vi "Broadcast.vi"   [LabVIEW 2015]
uses:
  Global/Globalclient.vi
types:
  T1 = enum16{"Standard", "Buffered", "CRLF", "Immediate"}
  T2 = typedef "消息头.ctl" = string[]
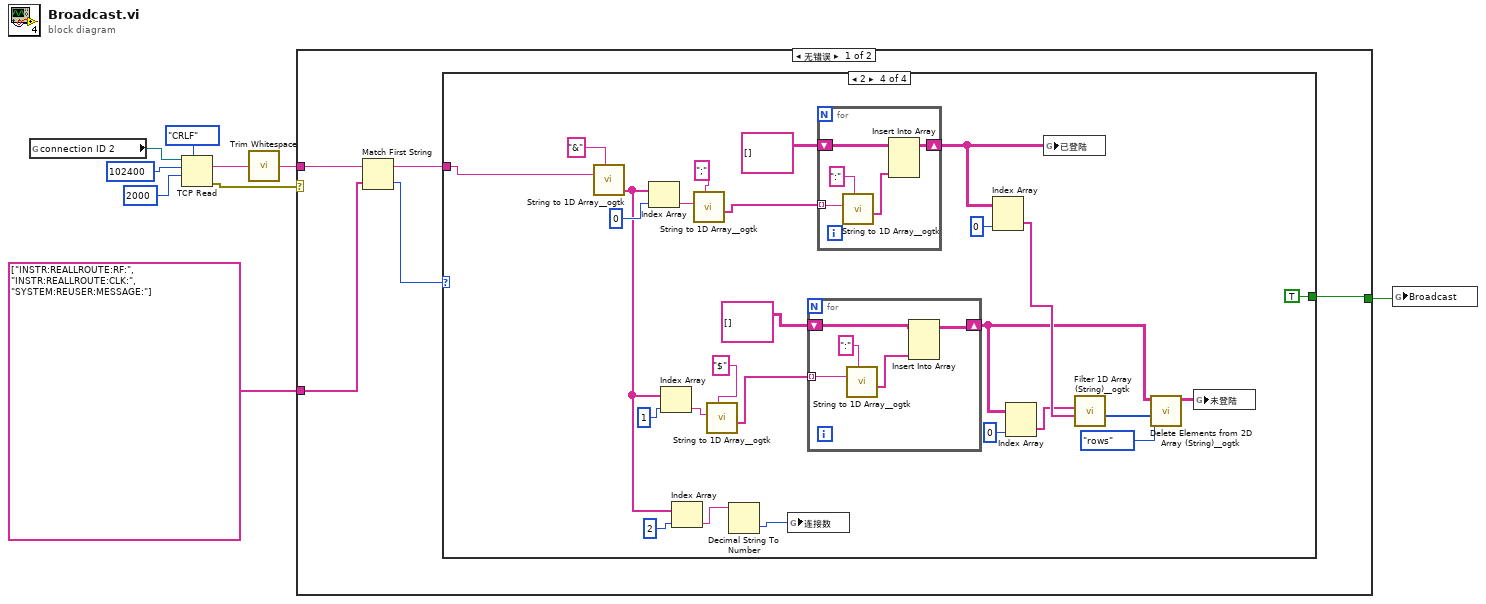
[diagram p0: block diagram]
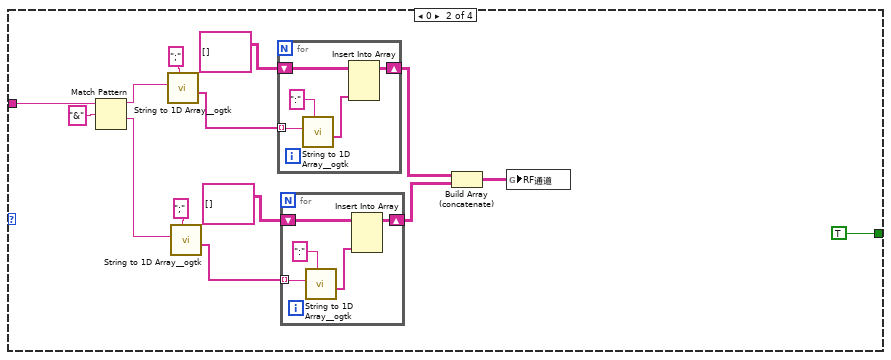
[diagram p3: hidden frame]
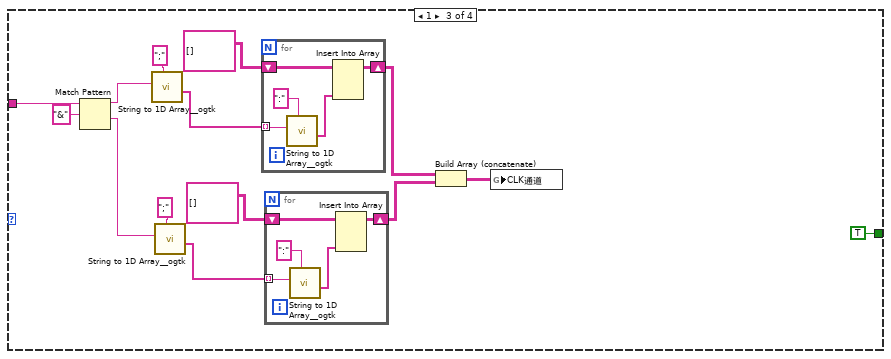
[diagram p4: hidden frame]
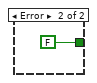
[diagram p5: hidden frame]
diagram:
  n1 = global read "Globalclient.vi" "connection ID 2"() -> (w9:refnum<k5>)
  n2 = TCP Read(connection ID=w9, bytes to read=102400, 7:T1."CRLF" ("mode (standard)"), 9:2000 ("timeout ms (25000)")) -> (data out=w3:string, error out=w4:errorcluster)  [unwired: 1 in, 1 out]
  n3 = call <vilib>:"Trim Whitespace.vi"("string"=w3) -> ("trimmed string"=w2:string)  [unwired: 1 in]
  n4 = case shown="无错误" w4 {
    tunnel: w2 -> [w14 _]
    tunnel: T2 ["INSTR:REALLROUTE:RF:", "INSTR:REALLROUTE:CLK:", "SYSTEM:REUSER:MESSAGE:"] ("消息头") -> [w13 _]
    tunnel: [w10 FALSE] -> w1
    frame No Error {
      n5 = Match First String(2:w13, 3:w14) -> (0:w11:i32, 1:w12:string)
      n6 = case shown="2" w11 {
        tunnel: w12 -> [_ w16 w41 w64]
        tunnel: [_ TRUE TRUE TRUE] -> w10
        frame Default {
        }
        frame 0 {
          n7 = Match Pattern(string=w16, regular expression="&") -> (before substring=w25:string, after substring=w19:string)  [unwired: 1 in, 2 out]
          n8 = call <userlib>:"String to 1D Array__ogtk.vi"("delimiter (Tab)"=";", "string"=w25) -> ("Array of Strings"=w24:string[])  [unwired: 9 in]
          n9 = call <userlib>:"String to 1D Array__ogtk.vi"("delimiter (Tab)"=";", "string"=w19) -> ("Array of Strings"=w21:string[])  [unwired: 9 in]
          n10 = for {
            tunnel: w24 -> [w38] mode=indexing
            shift-right: [w34] -> w18
            shift-left: string[][] [] -> [w36]
            n11 = call <userlib>:"String to 1D Array__ogtk.vi"("delimiter (Tab)"=":", "string"=w38) -> ("Array of Strings"=w35:string[])  [unwired: 9 in]
            n12 = Insert Into Array(array=w36, new element=w35) -> (w34:string[][])  [unwired: 2 in]
          }
          n13 = for {
            tunnel: w21 -> [w33] mode=indexing
            shift-right: [w29] -> w17
            shift-left: string[][] [] -> [w31]
            n14 = call <userlib>:"String to 1D Array__ogtk.vi"("delimiter (Tab)"=":", "string"=w33) -> ("Array of Strings"=w30:string[])  [unwired: 9 in]
            n15 = Insert Into Array(array=w31, new element=w30) -> (w29:string[][])  [unwired: 2 in]
          }
          n16 = Build Array (concatenate)(w18, w17) -> (w28:string[][])
          n17 = global write "Globalclient.vi" "RF通道"(w28) -> ()
        }
        frame 1 {
          n18 = Match Pattern(string=w41, regular expression="&") -> (before substring=w50:string, after substring=w44:string)  [unwired: 1 in, 2 out]
          n19 = call <userlib>:"String to 1D Array__ogtk.vi"("delimiter (Tab)"=";", "string"=w50) -> ("Array of Strings"=w49:string[])  [unwired: 9 in]
          n20 = call <userlib>:"String to 1D Array__ogtk.vi"("delimiter (Tab)"=";", "string"=w44) -> ("Array of Strings"=w46:string[])  [unwired: 9 in]
          n21 = for {
            tunnel: w49 -> [w62] mode=indexing
            shift-right: [w58] -> w43
            shift-left: string[][] [] -> [w60]
            n22 = call <userlib>:"String to 1D Array__ogtk.vi"("delimiter (Tab)"=":", "string"=w62) -> ("Array of Strings"=w59:string[])  [unwired: 9 in]
            n23 = Insert Into Array(array=w60, new element=w59) -> (w58:string[][])  [unwired: 2 in]
          }
          n24 = for {
            tunnel: w46 -> [w57] mode=indexing
            shift-right: [w53] -> w42
            shift-left: string[][] [] -> [w55]
            n25 = call <userlib>:"String to 1D Array__ogtk.vi"("delimiter (Tab)"=":", "string"=w57) -> ("Array of Strings"=w54:string[])  [unwired: 9 in]
            n26 = Insert Into Array(array=w55, new element=w54) -> (w53:string[][])  [unwired: 2 in]
          }
          n27 = Build Array (concatenate)(w43, w42) -> (w40:string[][])
          n28 = global write "Globalclient.vi" "CLK通道"(w40) -> ()
        }
        frame 2 {
          n29 = call <userlib>:"String to 1D Array__ogtk.vi"("delimiter (Tab)"="&", "string"=w64) -> ("Array of Strings"=w70:string[])  [unwired: 9 in]
          n30 = Index Array(array=w70, index=0) -> (element=w79:string)
          n31 = Index Array(array=w70, index=1) -> (element=w75:string)
          n32 = Index Array(array=w70, index=2) -> (element=w68:string)
          n33 = call <userlib>:"String to 1D Array__ogtk.vi"("delimiter (Tab)"=";", "string"=w79) -> ("Array of Strings"=w77:string[])  [unwired: 9 in]
          n34 = call <userlib>:"String to 1D Array__ogtk.vi"("delimiter (Tab)"="$", "string"=w75) -> ("Array of Strings"=w74:string[])  [unwired: 9 in]
          n35 = Decimal String To Number(string=w68) -> (number=w65:i32)  [unwired: 2 in, 1 out]
          n36 = global write "Globalclient.vi" "连接数"(w65) -> ()
          n37 = for {
            tunnel: w74 -> [w93] mode=indexing
            shift-right: [w89] -> w71
            shift-left: string[][] [] -> [w91]
            n38 = call <userlib>:"String to 1D Array__ogtk.vi"("delimiter (Tab)"=":", "string"=w93) -> ("Array of Strings"=w90:string[])  [unwired: 9 in]
            n39 = Insert Into Array(array=w91, new element=w90) -> (w89:string[][])  [unwired: 2 in]
          }
          n40 = for {
            tunnel: w77 -> [w98] mode=indexing
            shift-right: [w94] -> w67
            shift-left: string[][] [] -> [w96]
            n41 = call <userlib>:"String to 1D Array__ogtk.vi"("delimiter (Tab)"=":", "string"=w98) -> ("Array of Strings"=w95:string[])  [unwired: 9 in]
            n42 = Insert Into Array(array=w96, new element=w95) -> (w94:string[][])  [unwired: 2 in]
          }
          n43 = Index Array(array=w67, index (col)=0 ("disabled index (col)")) -> (element=w82:string[])  [unwired: 1 in]
          n44 = Index Array(array=w71, index (col)=0 ("disabled index (col)")) -> (element=w72:string[])  [unwired: 1 in]
          n45 = global write "Globalclient.vi" "已登陆"(w67) -> ()
          n46 = call <userlib>:"Filter 1D Array (String)__ogtk.vi"("items to filter"=w82, "array"=w72) -> ("filtered item indices"=w81:i32[])  [unwired: 4 in, 1 out]
          n47 = call <userlib>:"Delete Elements from 2D Array (String)__ogtk.vi"("delete (rows or columns)"=enum16{"rows", "columns"}."rows", "indices"=w81, "array"=w71) -> ("array w/ subset deleted"=w66:string[][])  [unwired: 7 in, 1 out]
          n48 = global write "Globalclient.vi" "未登陆"(w66) -> ()
        }
      }
    }
    frame Error {
    }
  }
  n49 = global write "Globalclient.vi" "Broadcast"(w1) -> ()
